vi "Testing FPGA built in.vi"(4 "bottom":i16, 6 "top":i16, 7 "Jump Table":dbl[](array[numeric]), 8 "error in":errorcluster, 9 "Doodle in":T2, 10 "background":picture, 11 "FPGA VI Reference In":T1) -> (0 "error out":errorcluster, 3 "FPGA VI Reference Out":T1)   [LabVIEW 2019]
uses:
  <vilib>/picture/picture.llb/imagedata.ctl
  TypeDefs/FPGA Reference.ctl
panel:
  in  "milliseconds to wait":u32(slide)=50 scale=0.0..200.0
  in  "Col":i32(slide)=150 scale=0.0..264.0
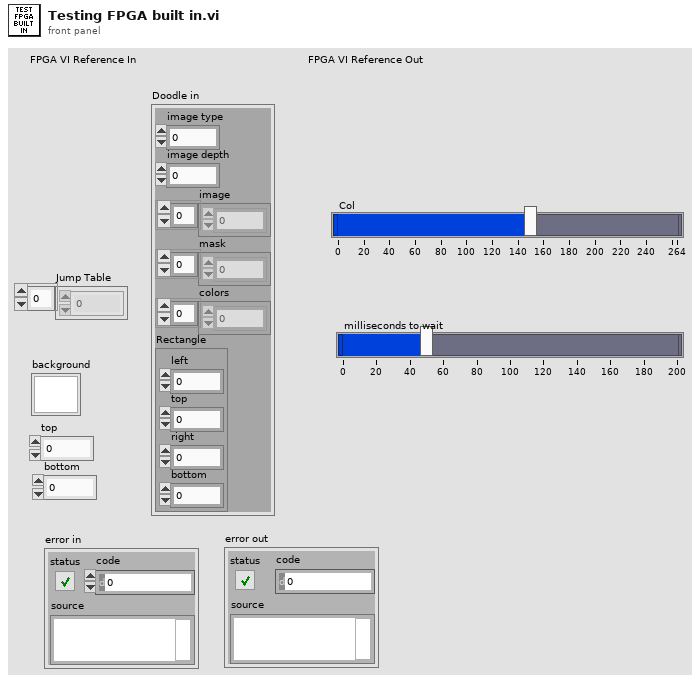
[diagram p1: front panel]
types:
  T1 = typedef "FPGA Reference.ctl" = refnum<k20>
  T2 = typedef "imagedata.ctl" = cluster{"image type":i32, "image depth":i32, "image":u8[], "mask":u8[], "colors":u32[], "Rectangle":cluster{"left":i16, "top":i16, "right":i16, "bottom":i16}}
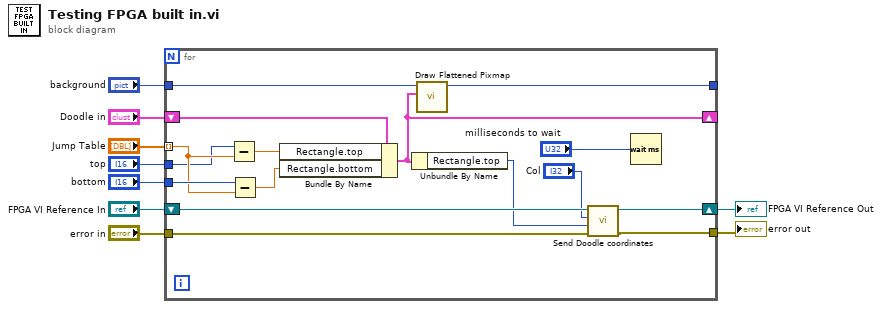
[diagram p0: block diagram]
diagram:
  n1 = for {
    tunnel: "Jump Table" -> [w21] mode=indexing
    tunnel: "top" -> [w20]
    tunnel: "bottom" -> [w22]
    shift-right: [w12] -> _
    shift-left: "Doodle in" -> [w25]
    tunnel: "background" -> [w18]
    tunnel: [w17] -> _
    tunnel: "error in" -> [w13]
    tunnel: [w14] -> w2
    shift-right: [w15] -> w1
    shift-left: "FPGA VI Reference In" -> [w16]
    n2 = Subtract(x=w20, y=w21) -> (x-y=w24:dbl)
    n3 = Subtract(x=w22, y=w21) -> (x-y=w23:dbl)
    n4 = Bundle By Name(cluster=w25, "Rectangle.top"=w24, "Rectangle.bottom"=w23) -> (w12:T2)
    n5 = Unbundle By Name(w12) -> ("Rectangle.top"=w10:i16)
    n6 = call <vilib>:"Draw Flattened Pixmap.vi"("image data"=w12, "picture"=w18) -> ("new picture"=w17:picture)  [unwired: 7 in]
    n7 = call "Send Doodle coordinates.vi"("error in"=w13, "Row"=w10, "Col"="Col", "FPGA VI Reference Out"=w16) -> ("error out"=w14:errorcluster, "FPGA VI Reference Out 2"=w15:T1)  [unwired: 6 in]
    n8 = Wait (ms)(milliseconds to wait="milliseconds to wait") -> ()  [unwired: 1 out]
  }
  "error out" <- w2
  "FPGA VI Reference Out" <- w1
